vi "Increment.vi"(8 "error in (no error)":errorcluster, 11 "Standard in":refnum<class "Standard.lvclass">) -> (0 "error out":errorcluster, 3 "Standard out":refnum<class "Standard.lvclass">)   [LabVIEW 2018, in "Standard.lvclass"]
uses:
  Standard.lvclass
  Standard.lvclass/Standard.ctl
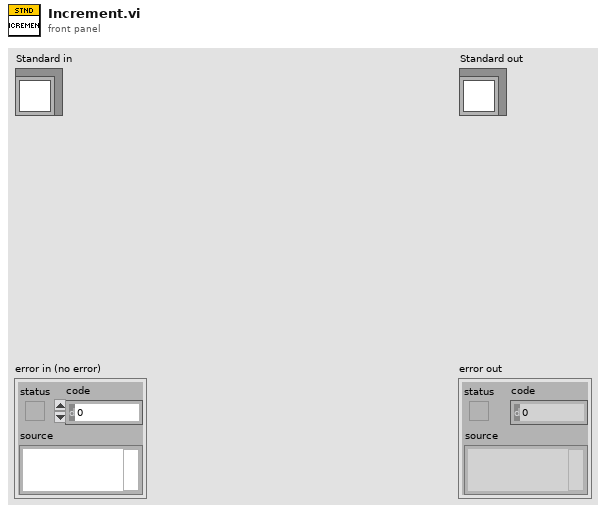
[diagram p1: front panel]
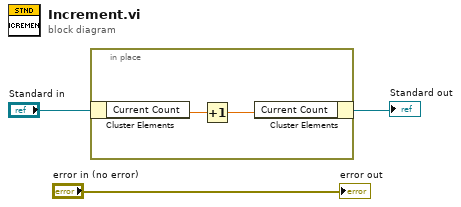
[diagram p0: block diagram]
diagram:
  n1 = in-place {
    n2 = in-place-cluster #1("Standard in") -> ("Current Count"=w5:cdb)
    n3 = Increment(x=w5) -> (x+1=w4:cdb)
    n4 = in-place-cluster #1("Current Count"=w4) -> (→"Standard out":refnum<class "Standard.lvclass">)
  }
  "error out" <- "error in (no error)"
